vi "Update Frame Element.vi"(9 "Detection Frame In in":refnum<class "Camera.lvclass">, 10 "Numeric":i32, 11 "Detection Frame in 3":refnum<class "Camera.lvclass">[](array[class])) -> (3 "Detection Frame in out":refnum<class "Camera.lvclass">[](array[class]))   [LabVIEW 2018]
uses:
  Camera_class/Camera.lvclass
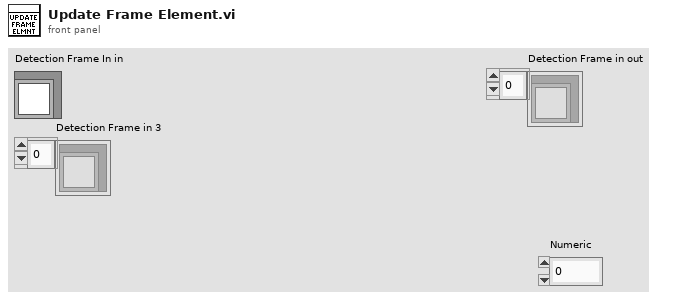
[diagram p1: front panel]
types:
  T1 = typedef "SSL Detection Robot.ctl" = cluster{"x":sgl, "robot_id":u32, "confidence":sgl, "y":sgl, "orientation":sgl, "pixel_x":sgl, "pixel_y":sgl, "height":sgl, "Valid":bool, "Time Stamp":timestamp, "x_k|k":T2, "Pk|k":T2, "Previous Time Stamp":timestamp, "R":T2}
  T2 = typedef "NI_Matrix.lvlib/RealMatrix.ctl" = dbl[][]
  T3 = typedef "SSL Detection Ball.ctl" = cluster{"x":sgl, "area":u32, "confidence":sgl, "y":sgl, "z":sgl, "pixel_x":sgl, "pixel_y":sgl, "Valid":bool, "Time Stamp":timestamp, "x_k|k":T2, "Pk|k":T2, "Id":u32, "Previous Time Stamp":timestamp, "R":T2}
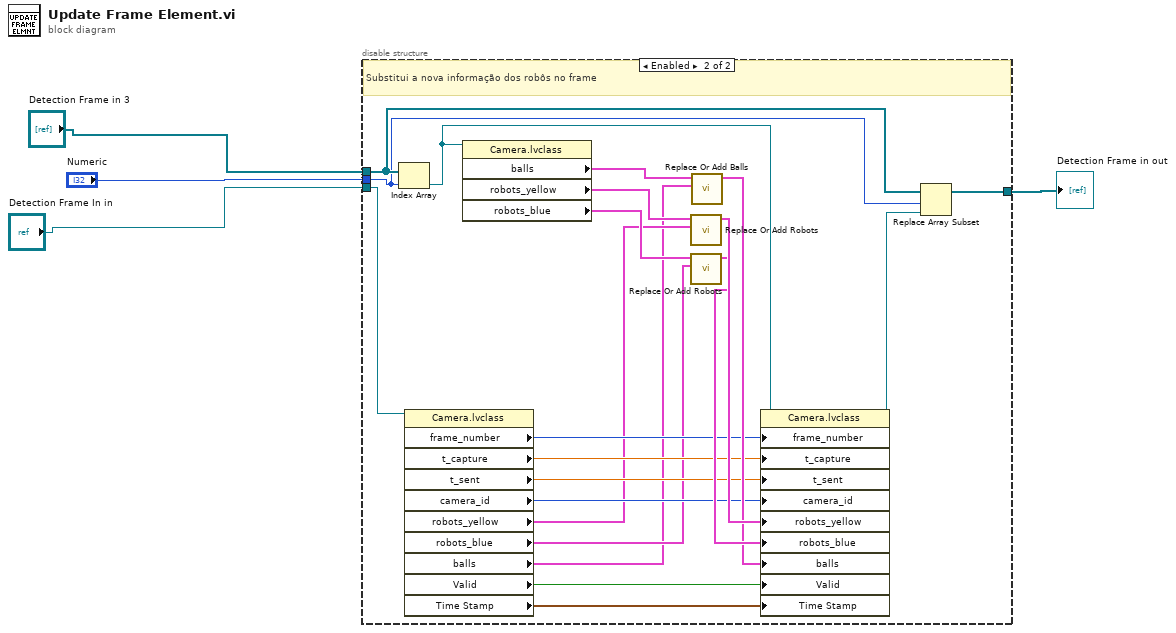
[diagram p0: block diagram]
diagram:
  n1 = disable-structure shown="Enabled" {
    disable-tunnel: "Detection Frame in 3" -> [_ w25]
    disable-tunnel: "Numeric" -> [_ w24]
    disable-tunnel: "Detection Frame In in" -> [_ w14]
    disable-tunnel: [_ w23] -> w1
    frame Disabled {
    }
    frame Enabled {
      # "Substitui a nova informação dos robôs no frame"
      n2 = Index Array(array=w25, index=w24) -> (element=w18:refnum<class "Camera.lvclass">)
      n3 = property class="Camera.lvclass"(reference=w14) -> ("frame_number"=w13:u32, "t_capture"=w12:dbl, "t_sent"=w11:dbl, "camera_id"=w10:u32, "robots_yellow"=w9:T1[], "robots_blue"=w8:T1[], "balls"=w7:T3[], "Valid"=w6:bool, "Time Stamp"=w5:timestamp)  [unwired: 1 in, 2 out]
      n4 = property class="Camera.lvclass"(reference=w18) -> ("balls"=w17:T3[], "robots_yellow"=w16:T1[], "robots_blue"=w15:T1[])  [unwired: 1 in, 2 out]
      n5 = call "Replace Or Add Robots.vi"("Robots New"=w9, "Robots Old"=w16) -> ("Robots New Out"=w21:T1[])  [unwired: 9 in]
      n6 = call "Replace Or Add Robots.vi"("Robots New"=w8, "Robots Old"=w15) -> ("Robots New Out"=w20:T1[])  [unwired: 9 in]
      n7 = call "Replace Or Add Balls.vi"("balls new"=w7, "balls"=w17) -> ("Balls out"=w19:T3[])  [unwired: 9 in]
      n8 = property class="Camera.lvclass"(reference=w18, "frame_number"=w13, "t_capture"=w12, "t_sent"=w11, "camera_id"=w10, "robots_yellow"=w21, "robots_blue"=w20, "balls"=w19, "Valid"=w6, "Time Stamp"=w5) -> (reference out=w22:refnum<class "Camera.lvclass">)  [unwired: 1 in, 1 out]
      n9 = Replace Array Subset(array=w25, new element=w22, index=w24) -> (w23:refnum<class "Camera.lvclass">[])
    }
  }
  "Detection Frame in out" <- w1
